vi "marshalling.vi"(8 "error in (no error)":errorcluster, 10 "Variant":variant, 11 "Serializer in":refnum<class "Serializer.erdosmiller-TOML.lvclass">) -> (0 "error out":errorcluster, 2 "String":string, 3 "Serializer":refnum<class "Serializer.erdosmiller-TOML.lvclass">)   [LabVIEW 2019, in "OpenSerializer.erdosmiller-TOML.lvlib" / "Serializer.erdosmiller-TOML.lvclass"]
uses:
  Serializer.erdosmiller-TOML.lvclass
  <vilib>/Erdos Miller/LV-TOML/LV-TOML.lvlib
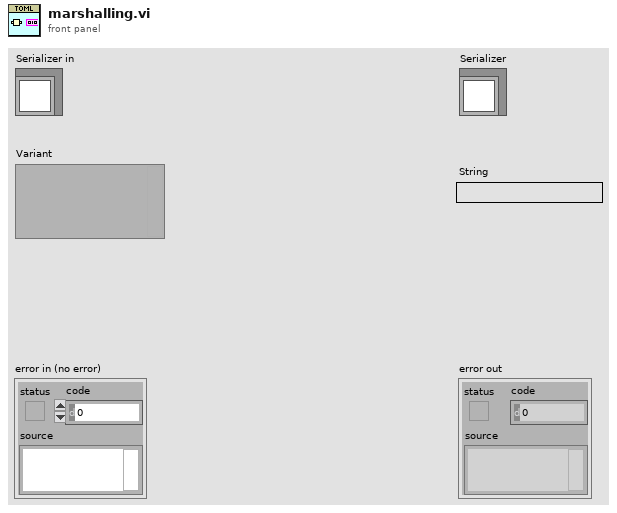
[diagram p1: front panel]
types:
  T1 = typedef "LV-TOML.lvlib/TOML Value.ctl" = cluster{"\\type":enum16{"Table", "Array", "String", "Integer", "Float", "Boolean", "Offset Date-Time", "Local Date-Time", "Local Date", "Local Time"}, "ÿýÿýÿýÿýÿýÿþÿýÿýÿý%LV-TOML.lvlib:TOML Key-Value Pair.ctlÿýÿýÿýÿýÿýÿþÿýÿýÿýLV-TOML.lvlib:TOML Value.ctl$":variant}
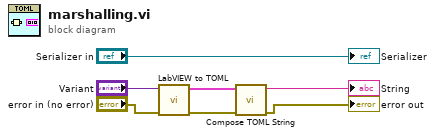
[diagram p0: block diagram]
diagram:
  n1 = call <vilib>:"LabVIEW to TOML.vi"("error in (no error)"="error in (no error)", "LV Value"="Variant") -> ("error out"=w4:errorcluster, "TOML Value"=w5:T1)  [unwired: 8 in]
  n2 = call <vilib>:"Compose TOML String.vi"("error in (no error)"=w4, "Value"=w5) -> ("error out"=→"error out":errorcluster, "String"=→"String":string)  [unwired: 8 in]
  "Serializer" <- "Serializer in"
